vi "ImageSend.vi"(2 "error in (no error)":errorcluster, 3 "mode (T=AutoAim, F=HotGoal)":bool) -> (0 "error out":errorcluster)   [LabVIEW 2014]
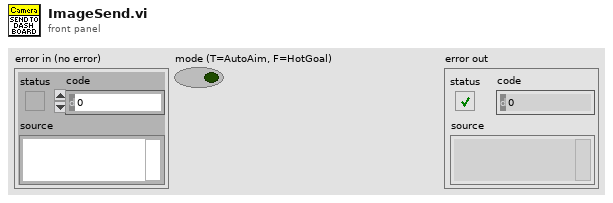
[diagram p1: front panel]
types:
  T1 = typedef "WPI_CameraDevRef.ctl" = cluster{"Camera Address":string, "CameraStatus":errorcluster, "Acquire Image Notifier":refnum<notifier>}
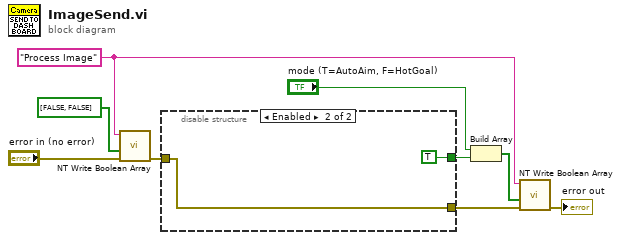
[diagram p0: block diagram]
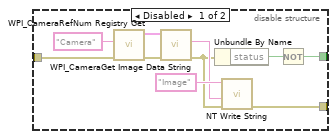
[diagram p2: hidden frame]
diagram:
  w2 = "Process Image" ("Name")
  n1 = call <vilib>:"NT Write Boolean Array.vi"("error in"="error in (no error)", "Boolean Array"=bool[] [FALSE, FALSE], "Name"=w2) -> ("error out"=w1:errorcluster)  [unwired: 8 in]
  n2 = disable-structure shown="Enabled" {
    disable-tunnel: [w17 w20] -> w9
    disable-tunnel: [w12 TRUE] -> w8
    disable-tunnel: w1 -> [w10 w20]
    frame Disabled {
      n3 = call <vilib>:"WPI_CameraRefNum Registry Get.vi"("error in (no error)"=w10, "refnum name"="Camera") -> ("error out"=w16:errorcluster, "CameraDevRef"=w15:T1)  [unwired: 8 in]
      n4 = call <vilib>:"WPI_CameraGet Image Data String.vi"("error in (no error)"=w16, "CameraDevRef"=w15) -> ("error out"=w11:errorcluster, "Image Data String"=w13:string)  [unwired: 7 in, 1 out]
      n5 = Unbundle By Name(w11) -> ("status"=w19:bool)
      n6 = call <vilib>:"NT Write String.vi"("error in"=w11, "String"=w13, "Name"="Image") -> ("error out"=w17:errorcluster)  [unwired: 8 in]
      n7 = Not(x=w19) -> (.not. x?=w12:bool)
    }
    frame Enabled {
    }
  }
  n8 = Build Array("mode (T=AutoAim, F=HotGoal)", w8) -> (w7:bool[])
  n9 = call <vilib>:"NT Write Boolean Array.vi"("error in"=w9, "Boolean Array"=w7, "Name"=w2) -> ("error out"=→"error out":errorcluster)  [unwired: 8 in]
